vi "Real-Time LED_Set Sequence.vi"(0 "Flash Period":i32, 5 "Sequence":bool[](array[boolean]), 7 "Color":enum8{"Off", "Green", "Amber"}(ring), 11 "error in (no error)":errorcluster) -> (14 "Roundtrip Time":dbl format="%.6fsec", 15 "error out":errorcluster)   [LabVIEW 2013]
uses:
  source/actor/Connector/FTW-ActorConnector.lvclass
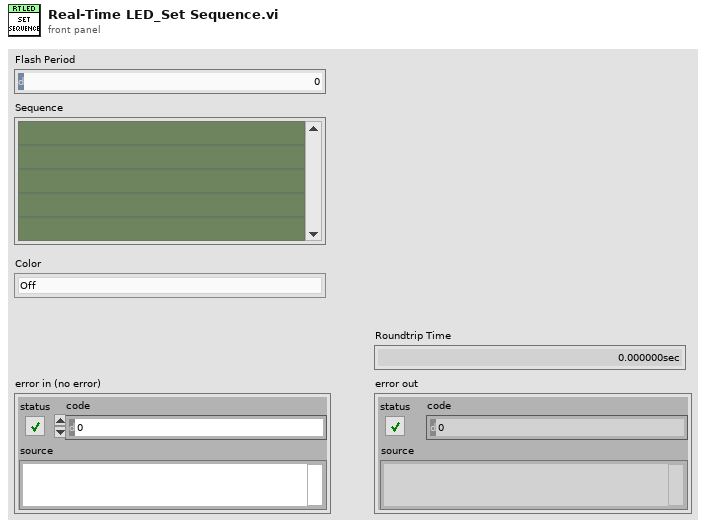
[diagram p1: front panel]
types:
  T1 = cluster{"Period":i32, "Sequence":bool[], "Color":i32}
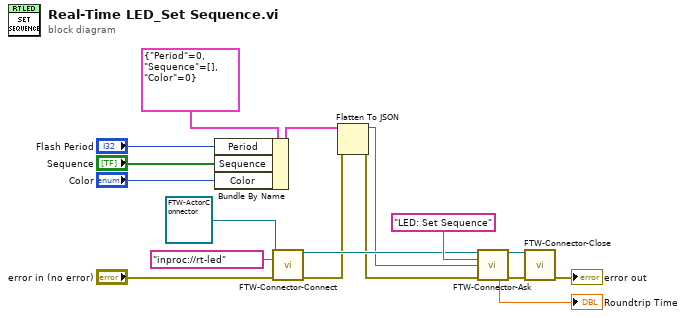
[diagram p0: block diagram]
diagram:
  n1 = Bundle By Name(cluster=T1 {"Period"=0, "Sequence"=[], "Color"=0}, "Period"="Flash Period", "Sequence"="Sequence", "Color"="Color") -> (w6:T1)
  n2 = call-dynamic "FTW-Connector-Connect.vi"("FTW Actor Connector Type"=refnum<class "FTW-ActorConnector.lvclass"> refnum, "Instance Inbox Address"="inproc://rt-led", "error in"="error in (no error)") -> ("FTW Actor Connector"=w12:refnum<class "FTW-ActorConnector.lvclass">, "error out"=w8:errorcluster)  [unwired: 11 in]
  n3 = Flatten To JSON(anything=w6, error in (no error)=w8) -> (JSON string=w1:string, 11:w7:errorcluster)  [unwired: 1 in]
  n4 = call "FTW-Connector-Ask.vi"("FTW Actor Connector"=w12, "Request Header"="LED: Set Sequence", "Request Body"=w1, "error in"=w7) -> ("FTW Actor Connector out"=w10:refnum<class "FTW-ActorConnector.lvclass">, "Roundtrip Time"=→"Roundtrip Time":dbl, "error out"=w15:errorcluster)  [unwired: 6 in, 3 out]
  n5 = call-dynamic "FTW-Connector-Close.vi"("FTW Actor Connector"=w10, "error in"=w15) -> ("error out"=→"error out":errorcluster)  [unwired: 13 in]
